vi "Create Serial Slave.vi"(4 "flow control":u16(ring) items=["None", "XON/XOFF", "RTS/CTS", "XON/XOFF & RTS/CTS", "DTR/DSR", "XON/XOFF & DTR/DSR"], 6 "parity (even)":u16(ring)=2 items=["None", "Odd", "Even", "Mark", "Space"], 7 "serial type":enum16{"RTU", "ASCII"}(ring), 8 "error in":errorcluster, 9 "Stop Bits(1.0)":u16(ring)=10 items=["1.0"=10, "1.5"=15, "2.0"=20], 10 "baud rate (9600)":u32=9600, 11 "VISA resource name":refnum<visa-resource-name>) -> (0 "error out":errorcluster, 3 "serial slave instance":refnum<class "Modbus Slave.lvclass">)   [LabVIEW 2013, in "Modbus Library - Advance.lvlib" / "API Main.lvlib"]
doc: "Creates a standard TCP slave with an IP ADU. If the data model input is unwired, a standard data model will be initialized and used. If the input is wired, the code will check to make sure that it is not the default value for the class (it should be initialized). If the default value of the class is wired, the standard model will be initialized and used."
uses:
  API Main.lvlib
  Slave/Modbus Slave.lvclass
  Transmission Data Unit/RTU/RTU Data Unit.lvclass
  Network Protocol/Network Slave/Serial/Serial Slave.lvclass
  Transmission Data Unit/ASCII/ASCII Data Unit.lvclass
  Modbus API.lvclass
  Transmission Data Unit/Transmission Data Unit.lvclass
  Super Data Model/Super Data Model.lvclass
panel:
  # "disable parity disallowed by mbspec"
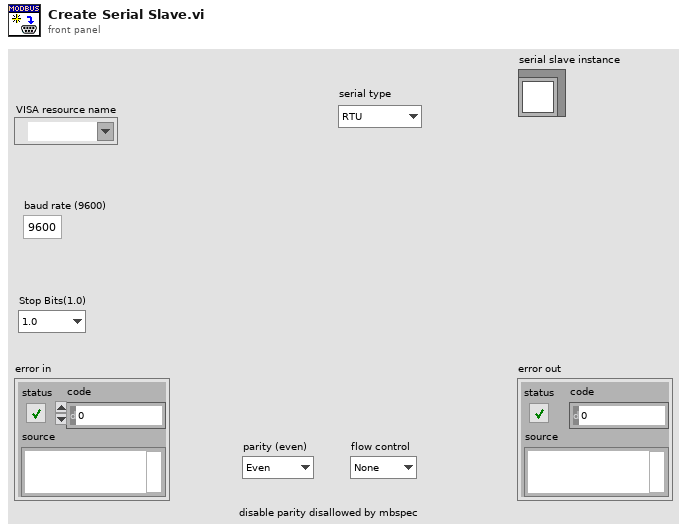
[diagram p1: front panel]
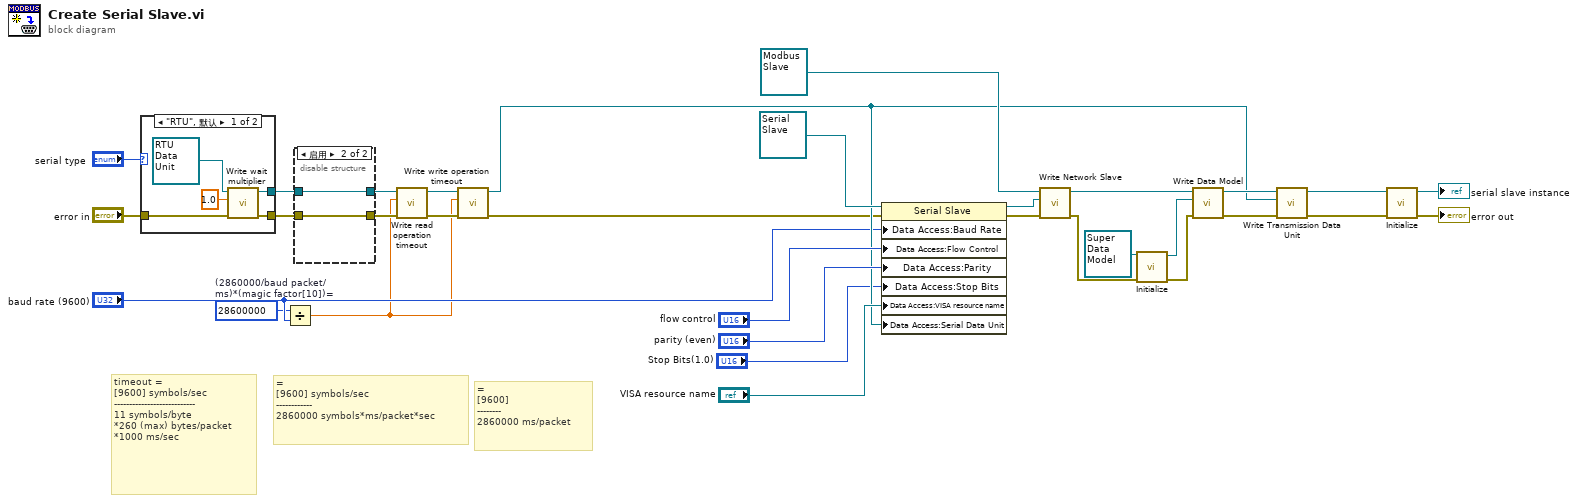
[diagram p0: block diagram]
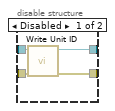
[diagram p2: hidden frame]
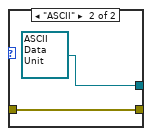
[diagram p3: hidden frame]
diagram:
  w11 = u32 28600000  # (2860000/baud packet/ms)*(magic factor[10])=
  # "=\n[9600]\n--------\n2860000 ms/packet"
  # "=\n[9600] symbols/sec\n------------\n2860000 symbols*ms/packet*sec"
  # "timeout =\n[9600] symbols/sec\n---------------------------\n11 symbols/byte\n*260 (max) bytes/packet\n*1000 ms/sec"
  n1 = case shown="\"RTU\", 默认" "serial type" {
    tunnel: [w37 w39] -> w9
    tunnel: "error in" -> [w36 w39]
    tunnel: [w33 refnum<class "ASCII Data Unit.lvclass"> refnum ("ASCII Data Unit")] -> w7
    frame "RTU", Default {
      n2 = call "Write wait multiplier.vi"("error in (no error)"=w36, "wait multiplier"=sgl 1.0, "RTU Data Unit in"=refnum<class "RTU Data Unit.lvclass"> refnum ("RTU Data Unit")) -> ("error out"=w37:errorcluster, "RTU Data Unit out"=w33:refnum<class "RTU Data Unit.lvclass">)  [unwired: 7 in]
    }
    frame "ASCII" {
    }
  }
  n3 = Divide(x=w11, y="baud rate (9600)") -> (x/y=w10:dbl)
  n4 = disable-structure shown="启用" {
    disable-tunnel: [w43 w45] -> w17
    disable-tunnel: [w42 w44] -> w13
    disable-tunnel: w9 -> [w41 w44]
    disable-tunnel: w7 -> [w40 w45]
    frame Disabled {
      n5 = call "Write Unit ID.vi"("error in"=w41, "transmission data unit in"=w40) -> ("error out"=w42:errorcluster, "transmission data unit out"=w43:refnum<class "Serial Data Unit.lvclass">)  [unwired: 8 in]
    }
    frame Enabled {
    }
  }
  n6 = call "Write read operation timeout.vi"("error in (no error)"=w13, "read operation timeout"=w10, "transmission data unit in"=w17) -> ("error out"=w14:errorcluster, "transmission data unit out"=w16:refnum<class "Serial Data Unit.lvclass">)  [unwired: 7 in]
  n7 = call "Write write operation timeout.vi"("error in (no error)"=w14, "write operation timeout"=w10, "transmission data unit in"=w16) -> ("error out"=w5:errorcluster, "transmission data unit out"=w15:refnum<class "Serial Data Unit.lvclass">)  [unwired: 7 in]
  n8 = property class="Serial Slave"(reference=refnum<class "Serial Slave.lvclass"> refnum ("Serial Slave"), error in=w5, "Data Access:Baud Rate"="baud rate (9600)", "Data Access:Flow Control"="flow control", "Data Access:Parity"="parity (even)", "Data Access:Stop Bits"="Stop Bits(1.0)", "Data Access:VISA resource name"="VISA resource name", "Data Access:Serial Data Unit"=w15) -> (reference out=w22:refnum<class "Serial Slave.lvclass">, error out=w21:errorcluster)
  n9 = call "Write Network Slave.vi"("error in"=w21, "network slave"=w22, "Modbus slave in"=refnum<class "Modbus Slave.lvclass"> refnum ("Modbus Slave")) -> ("error out"=w3:errorcluster, "Modbus slave out"=w20:refnum<class "Modbus Slave.lvclass">)  [unwired: 7 in]
  n10 = call "Initialize.vi"("错误输入（无错误）"=w3, "Super Data Model in"=refnum<class "Super Data Model.lvclass"> refnum) -> ("错误输出"=w4:errorcluster, "Super Data Model out"=w2:refnum<class "Super Data Model.lvclass">)  [unwired: 8 in]
  n11 = call "Write Data Model.vi"("error in"=w4, "Super Data Model"=w2, "Modbus slave in"=w20) -> ("error out"=w23:errorcluster, "Modbus slave out"=w24:refnum<class "Modbus Slave.lvclass">)  [unwired: 7 in]
  n12 = call "Write Transmission Data Unit.vi"("error in"=w23, "transmission data unit"=w15, "Modbus instance in"=w24) -> ("error out"=w25:errorcluster, "Modbus instance out"=w26:refnum<class "Modbus Slave.lvclass">)  [unwired: 7 in]
  n13 = call-dynamic "Initialize.vi"("error in"=w25, "Modbus slave in"=w26) -> ("error out"=→"error out":errorcluster, "Modbus slave out"=→"serial slave instance":refnum<class "Modbus Slave.lvclass">)  [unwired: 8 in]
